vi "getDistance_DriveQuadTalonSRX.vi"() -> (0 "Right Distance Ft":dbl format="%.4f", 3 "Left Distance FT":dbl format="%.4f")   [LabVIEW 2019, in "DriveQuadTalonSRX_Motor.lvlib"]
uses:
  DriveQuadTalonSRX_Motor.lvlib
  globals_DriveQuadTalonSRX.vi
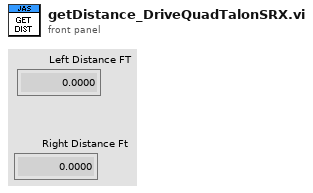
[diagram p1: front panel]
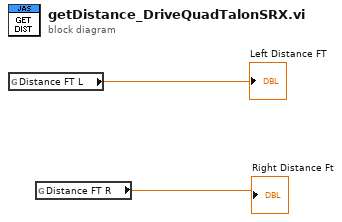
[diagram p0: block diagram]
diagram:
  n1 = global read "globals_DriveQuadTalonSRX.vi" "Distance FT L"() -> (→"Left Distance FT":dbl)
  n2 = global read "globals_DriveQuadTalonSRX.vi" "Distance FT R"() -> (→"Right Distance Ft":dbl)
